vi "UtilityLib.get unused TCP port Linux.vi"(2 "TCP port offset":u16, 5 "error in (no error)":errorcluster) -> (16 "TCP port":u16, 19 "error out":errorcluster)   [LabVIEW 2014, in "UtilityLib.lvlib"]
doc: "Obtains an unsed TCP port on the local machine. \n\nNote: This also works on Windows XP."
uses:
  UtilityLib.lvlib
panel:
  out "Ports in use":i32[](array[numeric])
  out "standard output":string
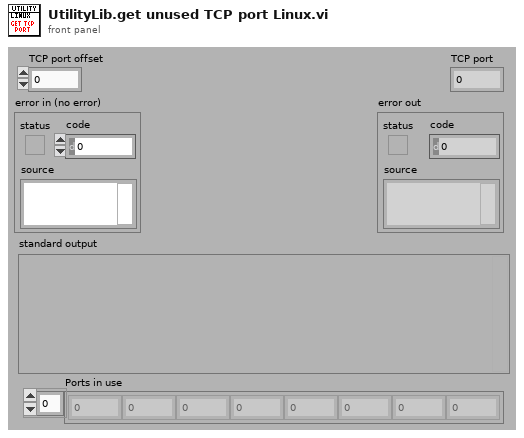
[diagram p1: front panel]
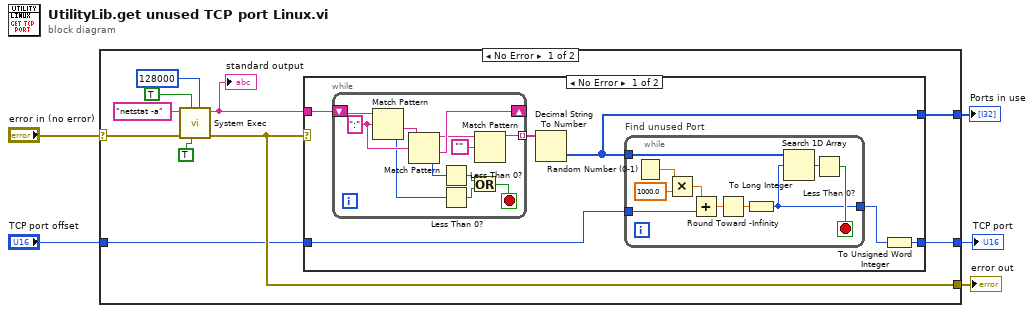
[diagram p0: block diagram]
diagram:
  n1 = case shown="No Error" "error in (no error)" {
    selector: "error in (no error)" -> [w11 w44]
    tunnel: [w10 w44] -> w4
    tunnel: "TCP port offset" -> [w8 _]
    tunnel: [w7 _] -> w2
    tunnel: [w6 _] -> w1
    frame No Error {
      n2 = call <vilib>:"System Exec.vi"("expected output size  (4096)"=u32 128000, "run minimized? (F)"=TRUE, "wait until completion? (T)"=TRUE, "error in (no error)"=w11, "command line"="netstat -a") -> ("error out"=w10:errorcluster, "standard output"=w12:string)  [unwired: 3 in, 2 out]
      "standard output" <- w12
      n3 = case shown="No Error" w10 {
        tunnel: w12 -> [w21 _]
        tunnel: w8 -> [w19 _]
        tunnel: [w18 _] -> w7
        tunnel: [w16 _] -> w6
        frame No Error {
          n4 = while {
            shift-right: [w41] -> _
            shift-left: w21 -> [w43]
            tunnel: [w33] -> w20 mode=indexing
            stop <- w32 stop-if-true
            w40 = ":" ("regular expression")
            n5 = Match Pattern(string=w43, regular expression=w40) -> (after substring=w42:string, offset past match=w39:i32)  [unwired: 1 in, 2 out]
            n6 = Match Pattern(string=w42, regular expression=w40) -> (before substring=w35:string, after substring=w41:string, offset past match=w38:i32)  [unwired: 1 in, 1 out]
            n7 = Less Than 0?(x=w38) -> (x < 0?=w37:bool)
            n8 = Less Than 0?(x=w39) -> (x < 0?=w36:bool)
            n9 = Or(x=w37, y=w36) -> (x .or. y?=w32:bool)
            n10 = Match Pattern(string=w35, regular expression="") -> (before substring=w33:string)  [unwired: 1 in, 3 out]
          }
          n11 = Decimal String To Number(string=w20) -> (number=w18:i32[])  [unwired: 2 in, 1 out]
          n12 = while "Find unused Port" {
            tunnel: w18 -> [w26]
            tunnel: [w23] -> w17
            tunnel: w19 -> [w22]
            stop <- w24 stop-if-true
            n13 = Random Number (0-1)() -> (number: 0 to 1=w31:dbl)
            n14 = Multiply(x=w31, y=1000.0) -> (x*y=w29:dbl)
            n15 = Add(x=w29, y=w22) -> (x+y=w28:dbl)
            n16 = Round Toward -Infinity ("Round To -Infinity")(1:w28) -> (0:w27:dbl)
            n17 = To Long Integer(number=w27) -> (32bit integer=w23:i32)
            n18 = Search 1D Array(1D array=w26, element=w23) -> (index of element=w25:i32)  [unwired: 1 in]
            n19 = Less Than 0?(x=w25) -> (x < 0?=w24:bool)
          }
          n20 = To Unsigned Word Integer(number=w17) -> (unsigned 16bit integer=w16:u16)
        }
        frame Error {
        }
      }
    }
    frame Error {
    }
  }
  "error out" <- w4
  "Ports in use" <- w2
  "TCP port" <- w1
